vi "GetDiagramReference.vi"(6 "error in":errorcluster, 9 "Diagram in":refnum<class "Diagram.lvclass">) -> (0 "error out":errorcluster, 1 "reference out":refnum<vi>, 3 "Diagram out":refnum<class "Diagram.lvclass">)   [LabVIEW 2014, in "Diagram.lvclass"]
uses:
  Diagram.lvclass
  Generic/Generic.lvclass
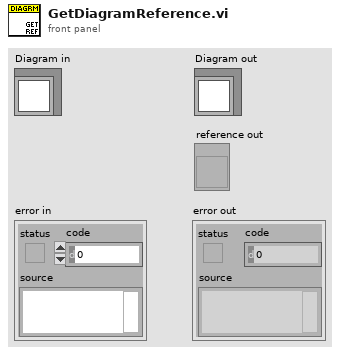
[diagram p1: front panel]
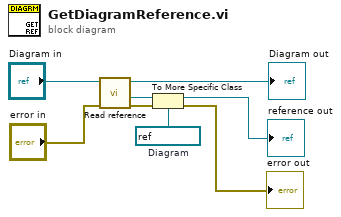
[diagram p0: block diagram]
diagram:
  w4 = refnum<vi> refnum  # Diagram
  n1 = call "Read reference.vi"("error in"="error in", "GObject in"="Diagram in") -> ("error out"=w5:errorcluster, "reference"=w6:refnum<vi>, "GObject out"=→"Diagram out":refnum<class "Diagram.lvclass">)  [unwired: 5 in]
  n2 = To More Specific Class(target class=w4, reference=w6, error in=w5) -> (specific class reference=→"reference out":refnum<vi>, error out=→"error out":errorcluster)
